vi "Decode UDP Message.vi"(11 "Input string":string) -> (3 "Data":T1={"Command"=enum."Speed", "Msg Length"=0, "Content"=[], "CRC8"=0, "Valid?"=FALSE})   [LabVIEW 2015]
uses:
  controls/UDP Message Data.ctl
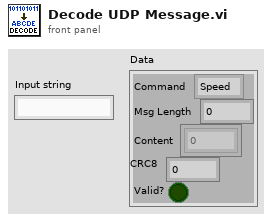
[diagram p1: front panel]
types:
  T1 = typedef "UDP Message Data.ctl" = cluster{"Command":enum16{"Acknowledge", "Speed", "Brake", "Watchdog", "Update", "Init", "Unknown"}, "Msg Length":u8, "Content":u8[], "CRC8":u8, "Valid?":bool}
  T2 = enum16{"Acknowledge", "Speed", "Brake", "Watchdog", "Update", "Init", "Unknown"}
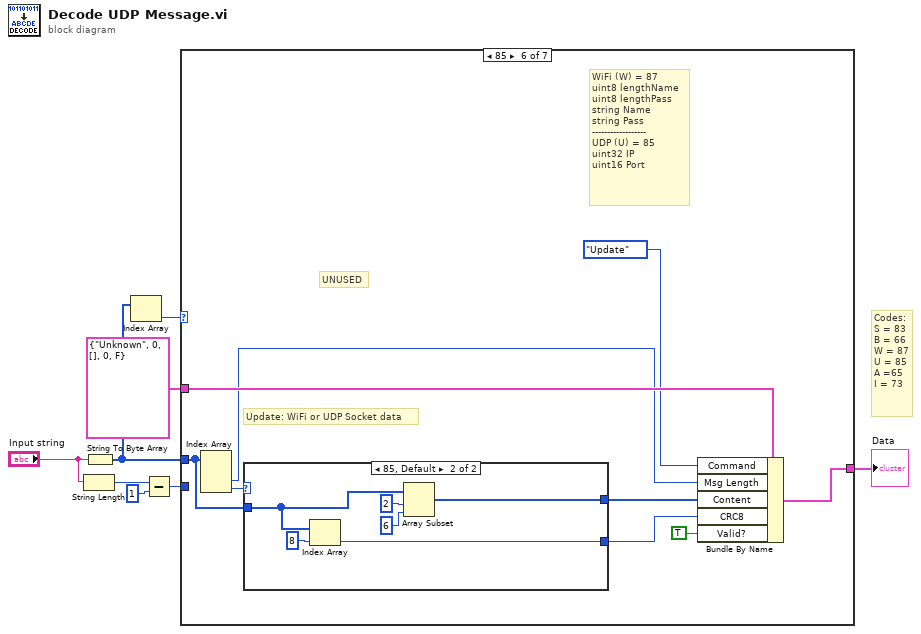
[diagram p0: block diagram]
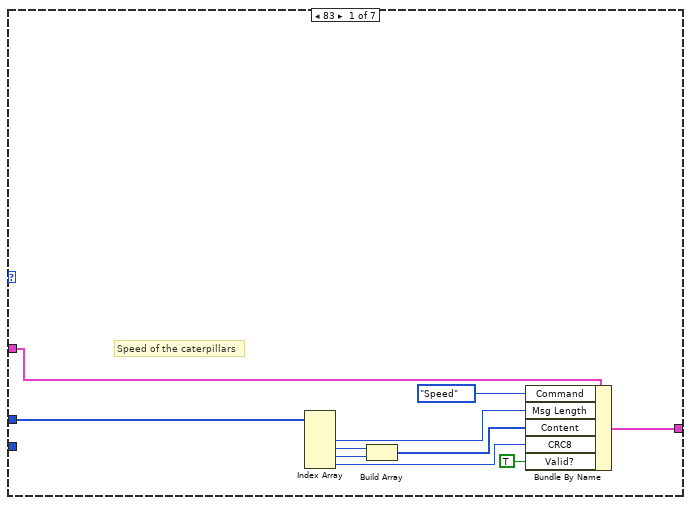
[diagram p2: hidden frame]
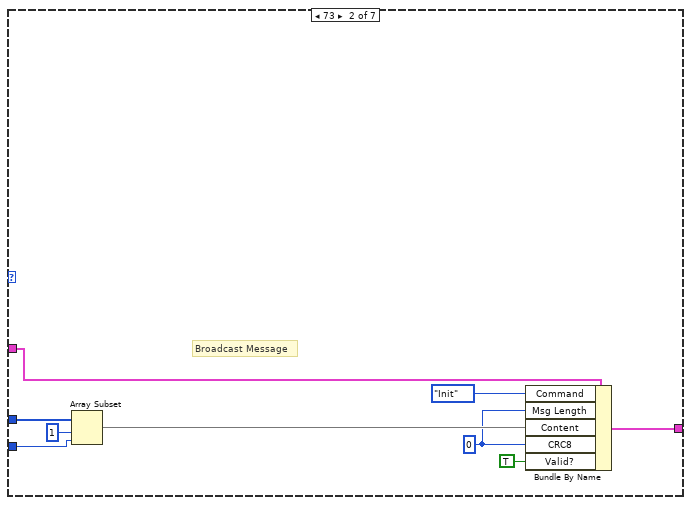
[diagram p3: hidden frame]
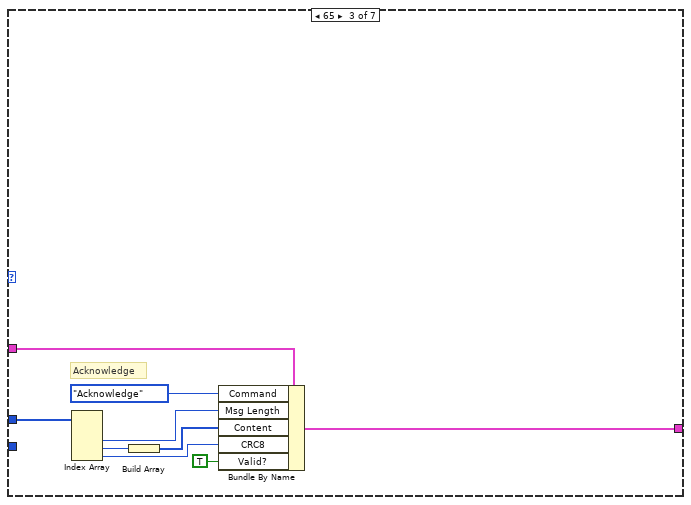
[diagram p4: hidden frame]
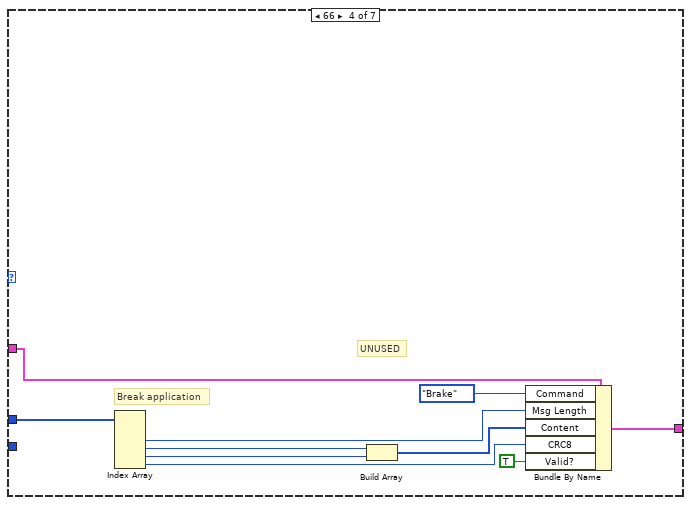
[diagram p5: hidden frame]
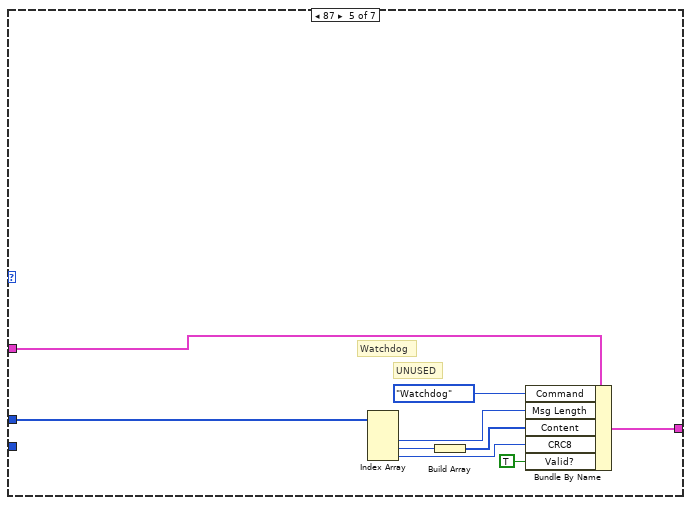
[diagram p6: hidden frame]
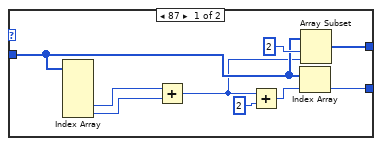
[diagram p7: hidden frame]
diagram:
  # "Codes:\nS = 83\nB = 66\nW = 87\nU = 85\nA =65\nI = 73"
  n1 = String Length(string="Input string") -> (length=w7:i32)
  n2 = String To Byte Array(string="Input string") -> (unsigned byte array=w1:u8[])
  n3 = Index Array(array=w1) -> (element=w2:u8)  [unwired: 1 in]
  n4 = Subtract(x=w7, y=1) -> (x-y=w5:i32)
  n5 = case shown="85" w2 {
    tunnel: w5 -> [_ w21 _ _ _ _ _]
    tunnel: T1 {"Command"=enum."Unknown", "Msg Length"=0, "Content"=[], "CRC8"=0, "Valid?"=FALSE} ("Data") -> [w18 w27 w36 w46 w55 w64 w80]
    tunnel: [w17 w26 w35 w45 w54 w63 w80] -> w4
    tunnel: w1 -> [w14 w23 w32 w43 w53 w60 _]
    frame 83 {
      # "Speed of the caterpillars"
      n6 = Index Array(array=w14) -> (element #2=w10:u8, element #3=w13:u8, element #4=w12:u8, element #5=w11:u8)  [unwired: 5 in, 1 out]
      n7 = Build Array(w13, w12) -> (w16:u8[])
      n8 = Bundle By Name(cluster=w18, "Command"=T2."Speed", "Msg Length"=w10, "Content"=w16, "CRC8"=w11, "Valid?"=TRUE) -> (w17:T1)
    }
    frame 73 {
      w19 = u8 0 ("Msg Length")
      # "Broadcast Message"
      n9 = Array Subset(array=w23, index=1, length=w21) -> (w20:u8[])
      n10 = Bundle By Name(cluster=w27, "Command"=T2."Init", "Msg Length"=w19, "Content"=w20, "CRC8"=w19, "Valid?"=TRUE) -> (w26:T1)
    }
    frame 65 {
      # "Acknowledge"
      n11 = Index Array(array=w32) -> (element #2=w30:u8, element #3=w31:u8, element #4=w29:u8)  [unwired: 4 in, 1 out]
      n12 = Build Array(w31) -> (w34:u8[])
      n13 = Bundle By Name(cluster=w36, "Command"=T2."Acknowledge", "Msg Length"=w30, "Content"=w34, "CRC8"=w29, "Valid?"=TRUE) -> (w35:T1)
    }
    frame 66 {
      # "UNUSED"
      # "Break application"
      n14 = Index Array(array=w43) -> (element #2=w38:u8, element #3=w41:u8, element #4=w42:u8, element #5=w39:u8)  [unwired: 5 in, 1 out]
      n15 = Build Array(w41, w42) -> (w40:u8[])
      n16 = Bundle By Name(cluster=w46, "Command"=T2."Brake", "Msg Length"=w38, "Content"=w40, "CRC8"=w39, "Valid?"=TRUE) -> (w45:T1)
    }
    frame 87 {
      # "UNUSED"
      # "Watchdog"
      n17 = Index Array(array=w53) -> (element #2=w48:u8, element #3=w52:u8, element #4=w50:u8)  [unwired: 4 in, 1 out]
      n18 = Build Array(w52) -> (w51:u8[])
      n19 = Bundle By Name(cluster=w55, "Command"=T2."Watchdog", "Msg Length"=w48, "Content"=w51, "CRC8"=w50, "Valid?"=TRUE) -> (w54:T1)
    }
    frame 85 {
      # "UNUSED"
      # "WiFi (W) = 87\nuint8 lengthName\nuint8 lengthPass\nstring Name\nstring Pass\n------------------\nUDP (U) = 85\nuint32 IP\nuint16 Port"
      # "Update: WiFi or UDP Socket data"
      n20 = Index Array(array=w60) -> (element #2=w57:u8, element #3=w59:u8)  [unwired: 3 in, 1 out]
      n21 = case shown="85, Default" w59 {
        tunnel: w60 -> [w72 w75]
        tunnel: [w68 w77] -> w62
        tunnel: [w71 w74] -> w61
        frame 87 {
          n22 = Index Array(array=w72) -> (element #4=w69:u8, element #5=w70:u8)  [unwired: 5 in, 3 out]
          n23 = Add(x=w69, y=w70) -> (x+y=w67:u8)
          n24 = Add(x=w67, y=u8 2) -> (x+y=w65:u8)
          n25 = Index Array(array=w72, index=w65) -> (element=w71:u8)
          n26 = Array Subset(array=w72, index=2, length=w67) -> (w68:u8[])
        }
        frame 85, Default {
          n27 = Index Array(array=w75, index=8 ("length")) -> (element=w74:u8)
          n28 = Array Subset(array=w75, index=2, length=6) -> (w77:u8[])
        }
      }
      n29 = Bundle By Name(cluster=w64, "Command"=T2."Update", "Msg Length"=w57, "Content"=w62, "CRC8"=w61, "Valid?"=TRUE) -> (w63:T1)
    }
    frame Default {
      # "Unknown"
    }
  }
  "Data" <- w4
